vi "test Add-Nonzero Bus Controller.vi"(8 "error in":errorcluster, 11 "TestCase in":refnum<class "Scripting.lvclass">) -> (0 "error out":errorcluster, 3 "TestCase out":refnum<class "Scripting.lvclass">)   [LabVIEW 2020, in "Scripting.lvclass"]
uses:
  Scripting.lvclass
  C:/Program Files (x86)/National Instruments/LabVIEW 2020/vi.lib/NI/VeriStand Custom Device Testing Tools/VeriStandScriptingTestCase/VeriStandScriptingTestCase.lvclass
  <vilib>/NI/VeriStand Custom Device Testing Tools/VeriStandScriptingTestCase/VeriStandScriptingTestCase.lvclass/VeriStandScriptingTestCase.ctl
  <vilib>/NI/VeriStand Custom Device Testing Tools/VeriStandScriptingTestCase/Read Target.vi
  NationalInstruments.VeriStand.SystemDefinitionAPI
  <vilib>/addons/_JKI Toolkits/VI Tester/TestCase.llb/TestCase.lvclass
  Scripting/Ballard MIL-STD-1553 Scripting.lvlib
  Shared/Address.ctl
  C:/Program Files (x86)/National Instruments/LabVIEW 2020/vi.lib/addons/_JKI Toolkits/VI Tester/TestCase.llb/TestCase.lvclass
  C:/dev/git/niveristand-ballard-milStd1553-custom-device/Source/Custom Device Support/Tests/Unit/Scripting/Scripting.lvclass
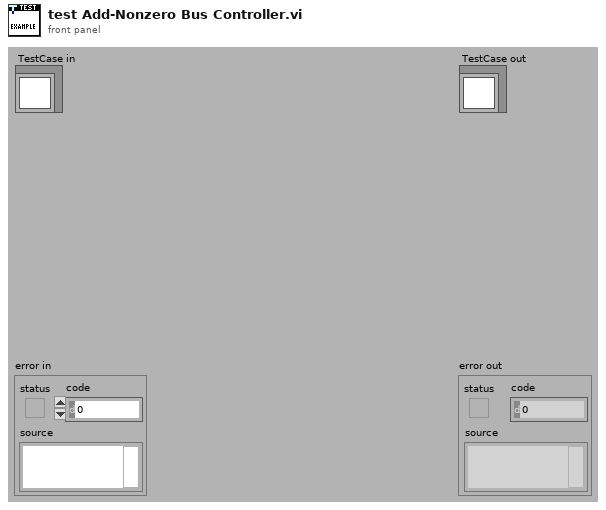
[diagram p1: front panel]
types:
  T1 = typedef "Address.ctl" = u16
  T2 = typedef "Custom Device API.lvlib/Custom Device Item Ref.ctl" = u64
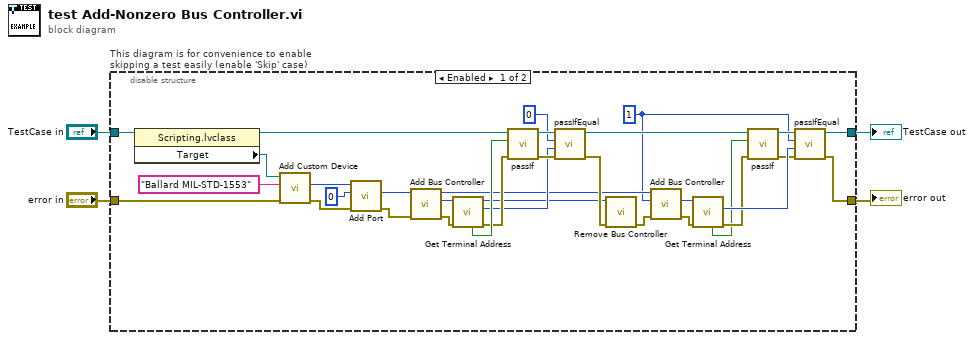
[diagram p0: block diagram]
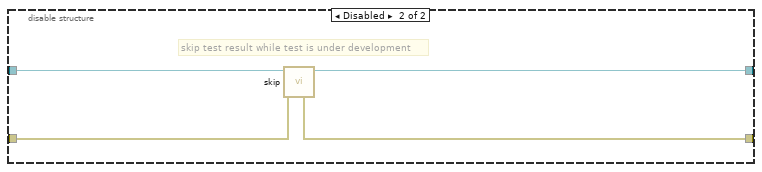
[diagram p2: hidden frame]
diagram:
  n1 = disable-structure "This diagram is for convenience to enable skipping a test easily (enable 'Skip' case)" shown="Enabled" {
    disable-tunnel: "TestCase in" -> [w35 w41]
    disable-tunnel: [w7 w39] -> w1
    disable-tunnel: [w18 w40] -> w3
    disable-tunnel: "error in" -> [w37 w38]
    frame Enabled {
      w5 = T1 1 ("terminal address (0)")
      n2 = property class="Scripting.lvclass"(reference=w35) -> (reference out=w29:refnum<class "Scripting.lvclass">, "Target"=w34:refnum<k24>)  [unwired: 1 in, 1 out]
      n3 = call "Add Custom Device.vi"("error in"=w37, "name"="Ballard MIL-STD-1553", "target in"=w34) -> ("error out"=w32:errorcluster, "Ballard MIL-STD 1553 custom device"=w31:T2)  [unwired: 6 in, 1 out]
      n4 = call "Add Port.vi"("error in"=w32, "port number"=u16 0, "Ballard MIL-STD 1553 custom device in"=w31) -> ("error out"=w30:errorcluster, "port"=w28:T2)  [unwired: 6 in, 1 out]
      n5 = call "Add Bus Controller.vi"("error in"=w30, "port in"=w28) -> ("error out"=w26:errorcluster, "bus controller"=w27:T2, "port out"=w8:T2)  [unwired: 7 in]
      n6 = call "Get Terminal Address.vi"("error in"=w26, "terminal in"=w27) -> ("error out"=w22:errorcluster, "terminal address"=w21:T1, "terminal out"=w9:T2, "found?"=w25:bool)  [unwired: 6 in]
      n7 = call-dynamic "passIf.vi"("error in (no error)"=w22, "pass"=w25, "TestCase in"=w29) -> ("error out"=w23:errorcluster, "TestCase out"=w24:refnum<class "Scripting.lvclass">)  [unwired: 7 in]
      n8 = call-dynamic "passIfEqual.vi"("error in (no error)"=w23, "y"=w21, "x"=T1 0 ("terminal address"), "TestCase in"=w24) -> ("error out"=w19:errorcluster, "TestCase out"=w6:refnum<class "Scripting.lvclass">)  [unwired: 6 in]
      n9 = call "Remove Bus Controller.vi"("error in"=w19, "bus controller"=w9) -> ("error out"=w10:errorcluster)  [unwired: 9 in]
      n10 = call "Add Bus Controller.vi"("error in"=w10, "terminal address (0)"=w5, "port in"=w8) -> ("error out"=w12:errorcluster, "bus controller"=w11:T2)  [unwired: 6 in, 1 out]
      n11 = call "Get Terminal Address.vi"("error in"=w12, "terminal in"=w11) -> ("error out"=w16:errorcluster, "terminal address"=w17:T1, "found?"=w13:bool)  [unwired: 6 in, 1 out]
      n12 = call-dynamic "passIf.vi"("error in (no error)"=w16, "pass"=w13, "TestCase in"=w6) -> ("error out"=w15:errorcluster, "TestCase out"=w14:refnum<class "Scripting.lvclass">)  [unwired: 7 in]
      n13 = call-dynamic "passIfEqual.vi"("error in (no error)"=w15, "y"=w17, "x"=w5, "TestCase in"=w14) -> ("error out"=w18:errorcluster, "TestCase out"=w7:refnum<class "Scripting.lvclass">)  [unwired: 6 in]
    }
    frame Disabled {
      # "skip test result while test is under development"
      n14 = call <vilib>:"skip.vi"("error in (no error)"=w38, "TestCase in"=w41) -> ("error out"=w40:errorcluster, "TestCase out"=w39:refnum<class "Scripting.lvclass">)  [unwired: 8 in]
    }
  }
  "error out" <- w3
  "TestCase out" <- w1
